vi "R1SBRControl_SetParams.vi"(7 "LabVIEW Web Service Request":refnum<class "Web Request.lvclass">, 11 "SetParams":T1) -> (2 "SBR_SetParams_out":T1, 3 "ControlStatus":string)   [LabVIEW 2016]
uses:
  <vilib>/wsapi/Web Request.lvclass
  Controls/R1SBR_SetParams.ctl
panel:
  # "Use the Web Service Request input terminal to call the VIs on the Web Services palette. Do not remove it from the connector pane unless you don't need access to the palette."
  # "Each additional control wired to the connector pane will be available as an input in the URL. To include an indicator in terminal-mode output (the default setting), it must also be wired to the connector pane."
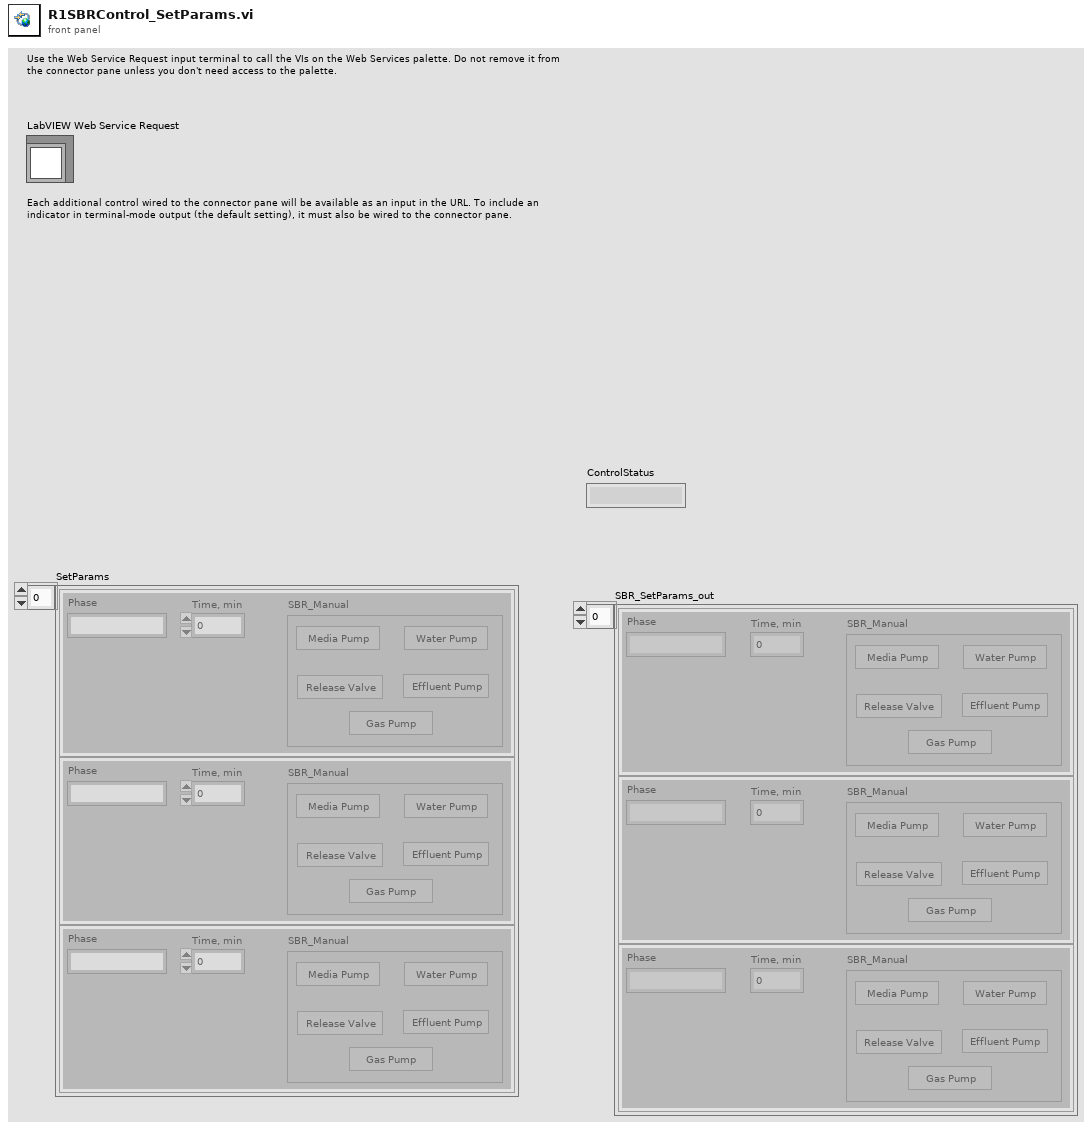
[diagram p1: front panel]
types:
  T1 = typedef "R1SBR_SetParams.ctl" = cluster{"Phase":string, "Time, min":dbl, "SBR_Manual":cluster{"Media Pump":bool, "Water Pump":bool, "Effluent Pump":bool, "Release Valve":bool, "Gas Pump":bool}}[]
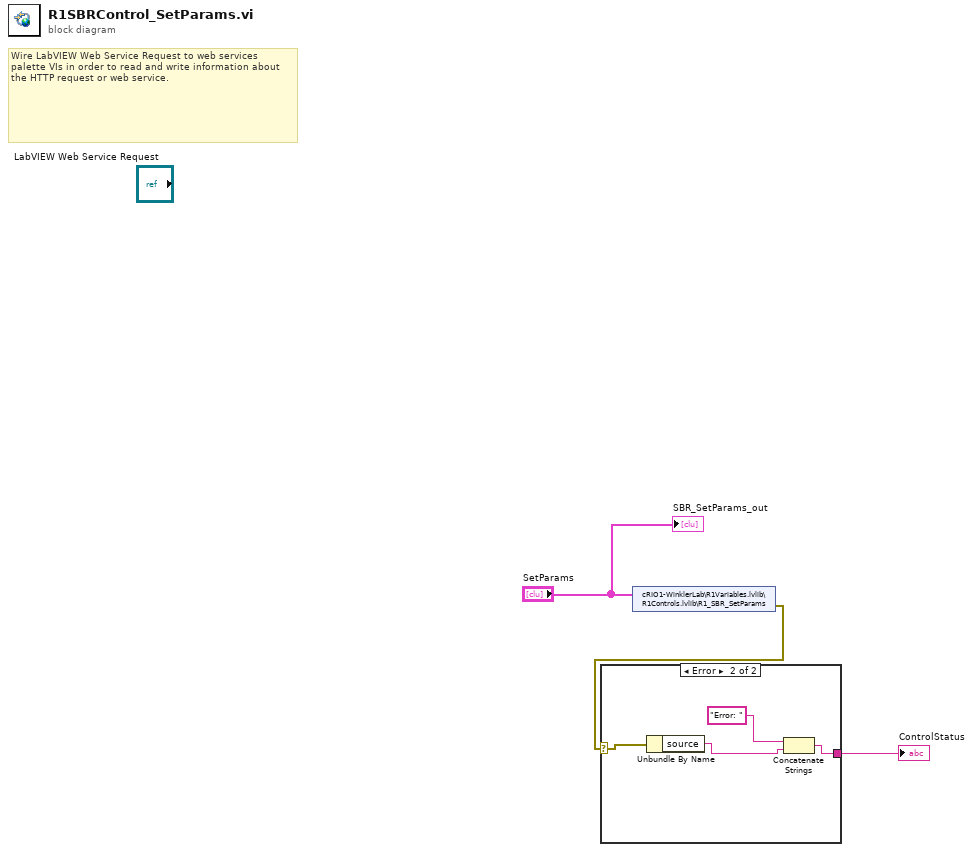
[diagram p0: block diagram]
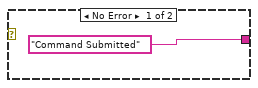
[diagram p2: hidden frame]
diagram:
  # "Wire LabVIEW Web Service Request to web services palette VIs in order to read and write information about the HTTP request or web service."
  n1 = shared-variable "cRIO1-WinklerLab\\R1Variables.lvlib\\R1Controls.lvlib\\R1_SBR_SetParams"("SetParams") -> (error out=w2:errorcluster)  [unwired: 1 in]
  n2 = case shown="Error" w2 {
    selector: w2 -> [_ w8]
    tunnel: ["Command Submitted" ("ControlStatus") w5] -> w1
    frame No Error {
    }
    frame Error {
      n3 = Unbundle By Name(w8) -> ("source"=w6:string)
      n4 = Concatenate Strings("Error: ", w6) -> (w5:string)
    }
  }
  "ControlStatus" <- w1
  "SBR_SetParams_out" <- "SetParams"
